vi "Dashboard Loop.VI"(7 "connection ID":refnum<k16>) -> ()   [LabVIEW 2015]
uses:
  Common Code/Dashboard Communication/Dashboard Display Data.ctl
  Common Code/Auton Command Cluster.ctl
  Common Code/Auton File Lists.ctl
  Common Code/Drivetrain Status Cluster.ctl
  Common Code/Drivetrain Modes.ctl
  Common Code/Dist Drive Status.ctl
  Common Code/Encoder Values Super Cluster.ctl
  Common Code/Encoder Values.ctl
  Common Code/IMU Data.ctl
  navX-MXP Library/COMMON/TypeDefs/Value TypeDefs/navX NAVX_CAL_STATUS.ctl
  navX-MXP Library/COMMON/TypeDefs/Value TypeDefs/navX NAVX_OP_STATUS.ctl
  Common Code/Power and Diagnostic Data.ctl
  Common Code/Utilities/PDP Data.ctl
  Common Code/Utilities/PCM Data.ctl
  Common Code/Shooter State Cluster.ctl
  Common Code/Shooter State.ctl
  Common Code/Shoot Modes Enum.ctl
  Common Code/Shot Type.ctl
  Common Code/Intake Status Cluster.ctl
  Common Code/Intake Mode.ctl
  Common Code/Intake States.ctl
  Common Code/Ultrasonic Data.ctl
  Common Code/Climb Status Cluster.ctl
  Common Code/Major Loop Times.ctl
  Robot Global Data.vi
  navX-MXP Library/navX-MXP IMU.lvlib
panel:
  out "Length":dbl
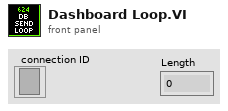
[diagram p1: front panel]
types:
  T1 = typedef "Major Loop Times.ctl" = cluster{"DT Loop Timer":u32, "Shooter Loop Timer":u32, "Intake Loop Timer":u32, "US Loop Timer":u32, "Auton File Loop Timer":u32}
  T2 = typedef "Dashboard Display Data.ctl" = cluster{"Auton Command Cluster":T3, "Auton File Lists":T4, "Drivetrain Status Cluster":T5, "Encoder Values":T8, "IMU Data":T10, "Power and Diagnostic Data":T13, "Gyro":dbl, "Shooter State Cluster":T16, "Intake Status Cluster":T20, "Ultrasonic Data":T23, "Climb Status Cluster":T24, "Loop Times":T1}
  T3 = typedef "Auton Command Cluster.ctl" = cluster{"Command ID":i32, "maxTime":dbl, "Y Distance":dbl, "Heading":dbl, "Throttle":dbl, "Async":dbl, "Velocity":dbl, "Acceleration":dbl, "To":dbl, "Condition":dbl, "Shot Type":dbl, "Left RPM":dbl, "Override RPM":i32, "Override Angle":i32, "Right RPM":dbl, "Angle":dbl, "Intake Mode":i32, "Intake Cmd":i32, "Intake O":i32, "Eject O":i32, "Angle O":i32, "Arm O":i32, "Intake Speed":dbl, "Eject Speed":dbl, "Arm Angle":dbl, "Arm Speed":dbl, "Intake?":i32, "Eject?":i32}
  T4 = typedef "Auton File Lists.ctl" = cluster{"Current Queue":string, "General Scripts":string, "Defense Scripts":string, "Movement Scripts":string}
  T5 = typedef "Drivetrain Status Cluster.ctl" = cluster{"Modes":T6, "Y (Throttle)":dbl, "X (Steer)":dbl, "Gyro In Range?":bool, "Distance Drive Finished?":bool, "Stop Eject Lockout":bool, "Dist Drive Status":T7, "Y Target":dbl, "Heading Target":dbl, "Vision Target Aligned?":bool, "Gear":dbl, "1st Gear Time":dbl, "2nd Gear Time":dbl, "1st Gear Shifts":dbl, "2nd Gear Shifts":dbl}
  T6 = typedef "Drivetrain Modes.ctl" = enum16{"Climb", "Manual", "Ball Vision Targeting", "Goal Vision Targeting", "PID Distance Drive", "Hybrid"}
  T7 = typedef "Dist Drive Status.ctl" = cluster{"Y In Range":bool, "X In Range":bool, "Gyro In Range":bool, "Y Dist":dbl, "X Dist":dbl, "Gyro":dbl}
  T8 = typedef "Encoder Values Super Cluster.ctl" = cluster{"Left Encoder":T9, "Right Encoder":T9}
  T9 = typedef "Encoder Values.ctl" = cluster{"Distance":dbl, "Speed":dbl, "Ticks":dbl}
  T10 = typedef "IMU Data.ctl" = cluster{"Pitch":sgl, "Roll":sgl, "Yaw":sgl, "Data Valid?":bool, "Temp":sgl, "MOVING":bool, "YAW_STABLE":bool, "Accel X":sgl, "Accel Y":sgl, "Accel Z":sgl, "Accel Magnitude":sgl, "Pitch Rate":sgl, "Roll Rate":sgl, "Yaw Rate":sgl, "NavX Opened?":bool, "NAVX_CAL_STATUS":T11, "NAVX_OP_STATUS":T12}
  T11 = typedef "navX-MXP IMU.lvlib/navX NAVX_CAL_STATUS.ctl" = u8
  T12 = typedef "navX-MXP IMU.lvlib/navX NAVX_OP_STATUS.ctl" = u8
  T13 = typedef "Power and Diagnostic Data.ctl" = cluster{"PDP Data":T14, "PCM Data":T15, "roboRIO input voltage (V)":dbl, "roboRIO input current (A)":dbl, "3.3V Rail Short":bool, "5 V Rail Short":bool, "6 V Rail Short":bool, "roboRIO Brownout":bool, "Outputs Enabled?":bool}
  T14 = typedef "PDP Data.ctl" = cluster{"Battery Voltage":sgl, "Temperature (degrees C)":sgl, "Internal Battery R (Ohms)":sgl, "Energy (J)":sgl, "Power (W)":sgl, "Total Current (A)":sgl, "Battery Voltage Fault":bool, "Temperature Fault":bool, "Hardware Fault":bool, "Currents":cluster{"[0]":sgl, "[1]":sgl, "[2]":sgl, "[3]":sgl, "[4]":sgl, "[5]":sgl, "[6]":sgl, "[7]":sgl, "[8]":sgl, "[9]":sgl, "[10]":sgl, "[11]":sgl, "[12]":sgl, "[13]":sgl, "[14]":sgl, "[15]":sgl}, "Current Faults":cluster{"[0]":bool, "[1]":bool, "[2]":bool, "[3]":bool, "[4]":bool, "[5]":bool, "[6]":bool, "[7]":bool, "[8]":bool, "[9]":bool, "[10]":bool, "[11]":bool, "[12]":bool, "[13]":bool, "[14]":bool, "[15]":bool}}
  T15 = typedef "PCM Data.ctl" = cluster{"Compressor Fault":bool, "Solenoid Fault":bool, "Compressor Enabled":bool, "Hardware Fault":bool, "Compressor Current":dbl}
  T16 = typedef "Shooter State Cluster.ctl" = cluster{"State":T17, "Left RPM":dbl, "Right RPM":dbl, "Shooter Ready?":bool, "Ball Loaded?":bool, "Current Angle":dbl, "Angle Motor Output":dbl, "Trigger Output":dbl, "Angle Ready?":bool, "RPM Ready?":bool, "Vision Ready?":bool, "Ball Loaded?":bool, "Mode":T18, "Shot Type":T19, "Pot Height":dbl, "Current Tripped Forward?":bool, "Current Tripped Backward?":bool, "Left Motor":dbl, "Right Motor":dbl, "Intake High?":bool, "Raw Left Pos":dbl, "Raw Right Pos":dbl, "Raw Left V":dbl, "Raw Right V":dbl, "Right Servo":i32, "Left Servo":i32}
  T17 = typedef "Shooter State.ctl" = enum16{"Idle", "Warmup", "Shooter Ready", "Shoot"}
  T18 = typedef "Shoot Modes Enum.ctl" = enum16{"Manual", "Safe", "Auto"}
  T19 = typedef "Shot Type.ctl" = enum16{"Batter Shot", "Corner Shot", "Curve Shot", "Vision Shot", "Deep Middle Shot"}
  T20 = typedef "Intake Status Cluster.ctl" = cluster{"Roller Power":dbl, "Angle Power":dbl, "Intake Mode":T21, "Intake States":T22, "Rollers Active?":bool, "Current Height":dbl, "Target Height":dbl, "Encoder Raw Position":dbl, "Forward Tripped?":bool, "Backward Tripped?":bool, "Override IR?":bool}
  T21 = typedef "Intake Mode.ctl" = enum16{"Safe", "Auto", "Manual"}
  T22 = typedef "Intake States.ctl" = enum16{"Idle", "Set roller speed", "Move to angle"}
  T23 = typedef "Ultrasonic Data.ctl" = cluster{"Left Ultrasonic":dbl, "Right Ultrasonic":dbl}
  T24 = typedef "Climb Status Cluster.ctl" = cluster{"Pull Power":dbl, "Unpin Power":dbl, "PTO Engaged?":bool, "Pull Height":dbl}
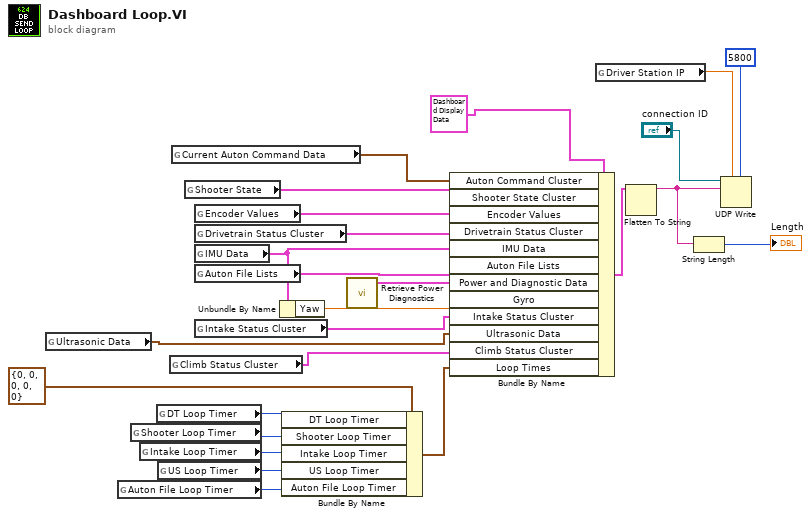
[diagram p0: block diagram]
diagram:
  n1 = global read "Robot Global Data.vi" "Ultrasonic Data"() -> (w8:T23)
  n2 = global read "Robot Global Data.vi" "Auton File Loop Timer"() -> (w2:u32)
  n3 = global read "Robot Global Data.vi" "Shooter Loop Timer"() -> (w5:u32)
  n4 = global read "Robot Global Data.vi" "Intake Loop Timer"() -> (w4:u32)
  n5 = global read "Robot Global Data.vi" "DT Loop Timer"() -> (w6:u32)
  n6 = global read "Robot Global Data.vi" "US Loop Timer"() -> (w3:u32)
  n7 = global read "Robot Global Data.vi" "Climb Status Cluster"() -> (w9:T24)
  n8 = global read "Robot Global Data.vi" "Current Auton Command Data"() -> (w20:T3)
  n9 = global read "Robot Global Data.vi" "Shooter State"() -> (w17:T16)
  n10 = global read "Robot Global Data.vi" "Encoder Values"() -> (w16:T8)
  n11 = global read "Robot Global Data.vi" "Drivetrain Status Cluster"() -> (w15:T5)
  n12 = global read "Robot Global Data.vi" "IMU Data"() -> (w12:T10)
  n13 = global read "Robot Global Data.vi" "Auton File Lists"() -> (w14:T4)
  n14 = global read "Robot Global Data.vi" "Intake Status Cluster"() -> (w10:T20)
  n15 = Unbundle By Name(w12) -> ("Yaw"=w11:sgl)
  n16 = Bundle By Name(cluster=T1 {"DT Loop Timer"=0, "Shooter Loop Timer"=0, "Intake Loop Timer"=0, "US Loop Timer"=0, "Auton File Loop Timer"=0} ("Loop Times"), "DT Loop Timer"=w6, "Shooter Loop Timer"=w5, "Intake Loop Timer"=w4, "US Loop Timer"=w3, "Auton File Loop Timer"=w2) -> (w1:T1)
  n17 = call "Retrieve Power Diagnostics.vi"() -> ("Power Cluster"=w13:T13)  [unwired: 11 in]
  n18 = Bundle By Name(cluster=T2 {"Auton Command Cluster"={"Command ID"=0, "maxTime"=0.0, "Y Distance"=0.0, "Heading"=0.0, "Throttle"=0.0, "Async"=0.0, "Velocity"=0.0, "Acceleration"=0.0, "To"=0.0, "Condition"=0.0, "Shot Type"=0.0, "Left RPM"=0.0, "Override RPM"=0, "Override Angle"=0, "Right RPM"=0.0, "Angle"=0.0, "Intake Mode"=0, "Intake Cmd"=0, "Intake O"=0, "Eject O"=0, "Angle O"=0, "Arm O"=0, "Intake Speed"=0.0, "Eject Speed"=0.0, "Arm Angle"=0.0, "Arm Speed"=0.0, "Intake?"=0, "Eject?"=0}, "Auton File Lists"={"Current Queue"="", "General Scripts"="", "Defense Scripts"="", "Movement Scripts"=""}, "Drivetrain Status Cluster"={"Modes"=enum."Manual", "Y (Throttle)"=0.0, "X (Steer)"=0.0, "Gyro In Range?"=FALSE, "Distance Drive Finished?"=FALSE, "Stop Eject Lockout"=FALSE, "Dist Drive Status"={"Y In Range"=FALSE, "X In Range"=FALSE, "Gyro In Range"=FALSE, "Y Dist"=0.0, "X Dist"=0.0, "Gyro"=0.0}, "Y Target"=0.0, "Heading Target"=0.0, "Vision Target Aligned?"=FALSE, "Gear"=0.0, "1st Gear Time"=0.0, "2nd Gear Time"=0.0, "1st Gear Shifts"=0.0, "2nd Gear Shifts"=0.0}, "Encoder Values"={"Left Encoder"={"Distance"=0.0, "Speed"=0.0, "Ticks"=0.0}, "Right Encoder"={"Distance"=0.0, "Speed"=0.0, "Ticks"=0.0}}, "IMU Data"={"Pitch"=0.0, "Roll"=0.0, "Yaw"=0.0, "Data Valid?"=FALSE, "Temp"=0.0, "MOVING"=FALSE, "YAW_STABLE"=FALSE, "Accel X"=0.0, "Accel Y"=0.0, "Accel Z"=0.0, "Accel Magnitude"=0.0, "Pitch Rate"=0.0, "Roll Rate"=0.0, "Yaw Rate"=0.0, "NavX Opened?"=FALSE, "NAVX_CAL_STATUS"=0, "NAVX_OP_STATUS"=0}, "Power and Diagnostic Data"={"PDP Data"={"Battery Voltage"=0.0, "Temperature (degrees C)"=0.0, "Internal Battery R (Ohms)"=0.0, "Energy (J)"=0.0, "Power (W)"=0.0, "Total Current (A)"=0.0, "Battery Voltage Fault"=FALSE, "Temperature Fault"=FALSE, "Hardware Fault"=FALSE, "Currents"={"[0]"=0.0, "[1]"=0.0, "[2]"=0.0, "[3]"=0.0, "[4]"=0.0, "[5]"=0.0, "[6]"=0.0, "[7]"=0.0, "[8]"=0.0, "[9]"=0.0, "[10]"=0.0, "[11]"=0.0, "[12]"=0.0, "[13]"=0.0, "[14]"=0.0, "[15]"=0.0}, "Current Faults"={"[0]"=FALSE, "[1]"=FALSE, "[2]"=FALSE, "[3]"=FALSE, "[4]"=FALSE, "[5]"=FALSE, "[6]"=FALSE, "[7]"=FALSE, "[8]"=FALSE, "[9]"=FALSE, "[10]"=FALSE, "[11]"=FALSE, "[12]"=FALSE, "[13]"=FALSE, "[14]"=FALSE, "[15]"=FALSE}}, "PCM Data"={"Compressor Fault"=FALSE, "Solenoid Fault"=FALSE, "Compressor Enabled"=FALSE, "Hardware Fault"=FALSE, "Compressor Current"=0.0}, "roboRIO input voltage (V)"=0.0, "roboRIO input current (A)"=0.0, "3.3V Rail Short"=FALSE, "5 V Rail Short"=FALSE, "6 V Rail Short"=FALSE, "roboRIO Brownout"=FALSE, "Outputs Enabled?"=FALSE}, "Gyro"=0.0, "Shooter State Cluster"={"State"=enum."Idle", "Left RPM"=0.0, "Right RPM"=0.0, "Shooter Ready?"=FALSE, "Ball Loaded?"=FALSE, "Current Angle"=0.0, "Angle Motor Output"=0.0, "Trigger Output"=0.0, "Angle Ready?"=FALSE, "RPM Ready?"=FALSE, "Vision Ready?"=FALSE, "Ball Loaded?"=FALSE, "Mode"=enum."Manual", "Shot Type"=enum."Batter Shot", "Pot Height"=0.0, "Current Tripped Forward?"=FALSE, "Current Tripped Backward?"=FALSE, "Left Motor"=0.0, "Right Motor"=0.0, "Intake High?"=FALSE, "Raw Left Pos"=0.0, "Raw Right Pos"=0.0, "Raw Left V"=0.0, "Raw Right V"=0.0, "Right Servo"=0, "Left Servo"=0}, "Intake Status Cluster"={"Roller Power"=0.0, "Angle Power"=0.0, "Intake Mode"=enum."Auto", "Intake States"=enum."Idle", "Rollers Active?"=FALSE, "Current Height"=0.0, "Target Height"=0.0, "Encoder Raw Position"=0.0, "Forward Tripped?"=FALSE, "Backward Tripped?"=FALSE, "Override IR?"=FALSE}, "Ultrasonic Data"={"Left Ultrasonic"=0.0, "Right Ultrasonic"=0.0}, "Climb Status Cluster"={"Pull Power"=0.0, "Unpin Power"=0.0, "PTO Engaged?"=FALSE, "Pull Height"=0.0}, "Loop Times"={"DT Loop Timer"=0, "Shooter Loop Timer"=0, "Intake Loop Timer"=0, "US Loop Timer"=0, "Auton File Loop Timer"=0}} ("Dashboard Status Data"), "Auton Command Cluster"=w20, "Shooter State Cluster"=w17, "Encoder Values"=w16, "Drivetrain Status Cluster"=w15, "IMU Data"=w12, "Auton File Lists"=w14, "Power and Diagnostic Data"=w13, "Gyro"=w11, "Intake Status Cluster"=w10, "Ultrasonic Data"=w8, "Climb Status Cluster"=w9, "Loop Times"=w1) -> (w19:T2)
  n19 = global read "Robot Global Data.vi" "Driver Station IP"() -> (w21:dbl)
  n20 = Flatten To String(anything=w19) -> (data string=w23:string)  [unwired: 3 in, 2 out]
  n21 = String Length(string=w23) -> (length=→"Length":i32)
  n22 = UDP Write(address=w21, port or service name=5800, connection ID="connection ID", data in=w23) -> ()  [unwired: 2 in, 2 out]
